vi "WILT.vi"() -> ()   [LabVIEW 2016] (continued)
            n368 = event-data() -> ("NewVal"=w742:bool)  [unwired: 1 in, 2 out]
            n369 = case shown="True" w742 {
              tunnel: w745 -> [_ w758]
              tunnel: w744 -> [w748 w756]
              tunnel: [w748 w755] -> w743
              tunnel: w742 -> [_ w753]
              frame False {
              }
              frame True {
                n370 = local read "Number of ON/OFF Cycles"() -> (w750:i32)
                n371 = local read "Valve ON Time (mS)"() -> (w749:u32)
                n372 = local read "Agilent Semaphore"() -> (w759:T1[])
                n373 = Unbundle By Name(w758) -> ("Agilent Switches"=w757:T2[])
                n374 = local read "Test Type"() -> (w751:T12)
                n375 = Number To Decimal String(number=32) -> (decimal integer string=w761:string)  [unwired: 1 in]
                n376 = Not(x=w753) -> (.not. x?=w760:bool)
                n377 = call "WILT Agilent Valve Control.vi"("Station In"=w761, "Agilent Channels In"=w757, "Semaphore"=w759, "Search"=T19 "Water Valve", "Open/Close (F:Close)"=w760, "error in (no error)"=w756, "Test Type"=w751, "Number Of Cycles"=w750, "Cycle Time (mS)"=w749) -> ("error out"=w755:errorcluster)  [unwired: 4 in, 2 out]
              }
            }
            n378 = call <vilib>:"Add State(s) to Queue__jki_lib_state_machine.vi"("State(s) in (\"\")"=w747) -> ("States Out"=w746:string)  [unwired: 14 in]
          }
          event Value Change {
            n379 = event-data() -> ("NewVal"=w762:bool)  [unwired: 1 in, 2 out]
            n380 = case shown="True" w762 {
              tunnel: w765 -> [_ w778]
              tunnel: w764 -> [w768 w776]
              tunnel: [w768 w775] -> w763
              tunnel: w762 -> [_ w773]
              frame False {
              }
              frame True {
                n381 = local read "Number of ON/OFF Cycles"() -> (w770:i32)
                n382 = local read "Valve ON Time (mS)"() -> (w769:u32)
                n383 = local read "Agilent Semaphore"() -> (w779:T1[])
                n384 = Unbundle By Name(w778) -> ("Agilent Switches"=w777:T2[])
                n385 = local read "Test Type"() -> (w771:T12)
                n386 = Number To Decimal String(number=33) -> (decimal integer string=w781:string)  [unwired: 1 in]
                n387 = Not(x=w773) -> (.not. x?=w780:bool)
                n388 = call "WILT Agilent Valve Control.vi"("Station In"=w781, "Agilent Channels In"=w777, "Semaphore"=w779, "Search"=T19 "Water Valve", "Open/Close (F:Close)"=w780, "error in (no error)"=w776, "Test Type"=w771, "Number Of Cycles"=w770, "Cycle Time (mS)"=w769) -> ("error out"=w775:errorcluster)  [unwired: 4 in, 2 out]
              }
            }
            n389 = call <vilib>:"Add State(s) to Queue__jki_lib_state_machine.vi"("State(s) in (\"\")"=w767) -> ("States Out"=w766:string)  [unwired: 14 in]
          }
          event Value Change {
            n390 = event-data() -> ("NewVal"=w782:bool)  [unwired: 1 in, 2 out]
            n391 = case shown="True" w782 {
              tunnel: w785 -> [_ w798]
              tunnel: w784 -> [w788 w796]
              tunnel: [w788 w795] -> w783
              tunnel: w782 -> [_ w793]
              frame False {
              }
              frame True {
                n392 = local read "Number of ON/OFF Cycles"() -> (w790:i32)
                n393 = local read "Valve ON Time (mS)"() -> (w789:u32)
                n394 = local read "Agilent Semaphore"() -> (w799:T1[])
                n395 = Unbundle By Name(w798) -> ("Agilent Switches"=w797:T2[])
                n396 = local read "Test Type"() -> (w791:T12)
                n397 = Number To Decimal String(number=34) -> (decimal integer string=w801:string)  [unwired: 1 in]
                n398 = Not(x=w793) -> (.not. x?=w800:bool)
                n399 = call "WILT Agilent Valve Control.vi"("Station In"=w801, "Agilent Channels In"=w797, "Semaphore"=w799, "Search"=T19 "Water Valve", "Open/Close (F:Close)"=w800, "error in (no error)"=w796, "Test Type"=w791, "Number Of Cycles"=w790, "Cycle Time (mS)"=w789) -> ("error out"=w795:errorcluster)  [unwired: 4 in, 2 out]
              }
            }
            n400 = call <vilib>:"Add State(s) to Queue__jki_lib_state_machine.vi"("State(s) in (\"\")"=w787) -> ("States Out"=w786:string)  [unwired: 14 in]
          }
          event Value Change {
            n401 = event-data() -> ("NewVal"=w802:bool)  [unwired: 1 in, 2 out]
            n402 = case shown="True" w802 {
              tunnel: w805 -> [_ w818]
              tunnel: w804 -> [w808 w816]
              tunnel: [w808 w815] -> w803
              tunnel: w802 -> [_ w813]
              frame False {
              }
              frame True {
                n403 = local read "Number of ON/OFF Cycles"() -> (w810:i32)
                n404 = local read "Valve ON Time (mS)"() -> (w809:u32)
                n405 = local read "Agilent Semaphore"() -> (w819:T1[])
                n406 = Unbundle By Name(w818) -> ("Agilent Switches"=w817:T2[])
                n407 = local read "Test Type"() -> (w811:T12)
                n408 = Number To Decimal String(number=35) -> (decimal integer string=w821:string)  [unwired: 1 in]
                n409 = Not(x=w813) -> (.not. x?=w820:bool)
                n410 = call "WILT Agilent Valve Control.vi"("Station In"=w821, "Agilent Channels In"=w817, "Semaphore"=w819, "Search"=T19 "Water Valve", "Open/Close (F:Close)"=w820, "error in (no error)"=w816, "Test Type"=w811, "Number Of Cycles"=w810, "Cycle Time (mS)"=w809) -> ("error out"=w815:errorcluster)  [unwired: 4 in, 2 out]
              }
            }
            n411 = call <vilib>:"Add State(s) to Queue__jki_lib_state_machine.vi"("State(s) in (\"\")"=w807) -> ("States Out"=w806:string)  [unwired: 14 in]
          }
          event Value Change {
            n412 = event-data() -> ("NewVal"=w822:bool)  [unwired: 1 in, 2 out]
            n413 = case shown="True" w822 {
              tunnel: w825 -> [_ w838]
              tunnel: w824 -> [w828 w836]
              tunnel: [w828 w835] -> w823
              tunnel: w822 -> [_ w833]
              frame False {
              }
              frame True {
                n414 = local read "Number of ON/OFF Cycles"() -> (w830:i32)
                n415 = local read "Valve ON Time (mS)"() -> (w829:u32)
                n416 = local read "Agilent Semaphore"() -> (w839:T1[])
                n417 = Unbundle By Name(w838) -> ("Agilent Switches"=w837:T2[])
                n418 = local read "Test Type"() -> (w831:T12)
                n419 = Number To Decimal String(number=36) -> (decimal integer string=w841:string)  [unwired: 1 in]
                n420 = Not(x=w833) -> (.not. x?=w840:bool)
                n421 = call "WILT Agilent Valve Control.vi"("Station In"=w841, "Agilent Channels In"=w837, "Semaphore"=w839, "Search"=T19 "Water Valve", "Open/Close (F:Close)"=w840, "error in (no error)"=w836, "Test Type"=w831, "Number Of Cycles"=w830, "Cycle Time (mS)"=w829) -> ("error out"=w835:errorcluster)  [unwired: 4 in, 2 out]
              }
            }
            n422 = call <vilib>:"Add State(s) to Queue__jki_lib_state_machine.vi"("State(s) in (\"\")"=w827) -> ("States Out"=w826:string)  [unwired: 14 in]
          }
          event Value Change {
            n423 = event-data() -> ("NewVal"=w842:bool)  [unwired: 1 in, 2 out]
            n424 = case shown="True" w842 {
              tunnel: w845 -> [_ w858]
              tunnel: w844 -> [w848 w856]
              tunnel: [w848 w855] -> w843
              tunnel: w842 -> [_ w853]
              frame False {
              }
              frame True {
                n425 = local read "Number of ON/OFF Cycles"() -> (w850:i32)
                n426 = local read "Valve ON Time (mS)"() -> (w849:u32)
                n427 = local read "Agilent Semaphore"() -> (w859:T1[])
                n428 = Unbundle By Name(w858) -> ("Agilent Switches"=w857:T2[])
                n429 = local read "Test Type"() -> (w851:T12)
                n430 = Number To Decimal String(number=37) -> (decimal integer string=w861:string)  [unwired: 1 in]
                n431 = Not(x=w853) -> (.not. x?=w860:bool)
                n432 = call "WILT Agilent Valve Control.vi"("Station In"=w861, "Agilent Channels In"=w857, "Semaphore"=w859, "Search"=T19 "Water Valve", "Open/Close (F:Close)"=w860, "error in (no error)"=w856, "Test Type"=w851, "Number Of Cycles"=w850, "Cycle Time (mS)"=w849) -> ("error out"=w855:errorcluster)  [unwired: 4 in, 2 out]
              }
            }
            n433 = call <vilib>:"Add State(s) to Queue__jki_lib_state_machine.vi"("State(s) in (\"\")"=w847) -> ("States Out"=w846:string)  [unwired: 14 in]
          }
          event Value Change {
            n434 = event-data() -> ("NewVal"=w862:bool)  [unwired: 1 in, 2 out]
            n435 = case shown="True" w862 {
              tunnel: w865 -> [_ w878]
              tunnel: w864 -> [w868 w876]
              tunnel: [w868 w875] -> w863
              tunnel: w862 -> [_ w873]
              frame False {
              }
              frame True {
                n436 = local read "Number of ON/OFF Cycles"() -> (w870:i32)
                n437 = local read "Valve ON Time (mS)"() -> (w869:u32)
                n438 = local read "Agilent Semaphore"() -> (w879:T1[])
                n439 = Unbundle By Name(w878) -> ("Agilent Switches"=w877:T2[])
                n440 = local read "Test Type"() -> (w871:T12)
                n441 = Number To Decimal String(number=38) -> (decimal integer string=w881:string)  [unwired: 1 in]
                n442 = Not(x=w873) -> (.not. x?=w880:bool)
                n443 = call "WILT Agilent Valve Control.vi"("Station In"=w881, "Agilent Channels In"=w877, "Semaphore"=w879, "Search"=T19 "Water Valve", "Open/Close (F:Close)"=w880, "error in (no error)"=w876, "Test Type"=w871, "Number Of Cycles"=w870, "Cycle Time (mS)"=w869) -> ("error out"=w875:errorcluster)  [unwired: 4 in, 2 out]
              }
            }
            n444 = call <vilib>:"Add State(s) to Queue__jki_lib_state_machine.vi"("State(s) in (\"\")"=w867) -> ("States Out"=w866:string)  [unwired: 14 in]
          }
          event Value Change {
            n445 = event-data() -> ("NewVal"=w882:bool)  [unwired: 1 in, 2 out]
            n446 = case shown="True" w882 {
              tunnel: w885 -> [_ w898]
              tunnel: w884 -> [w888 w896]
              tunnel: [w888 w895] -> w883
              tunnel: w882 -> [_ w893]
              frame False {
              }
              frame True {
                n447 = local read "Number of ON/OFF Cycles"() -> (w890:i32)
                n448 = local read "Valve ON Time (mS)"() -> (w889:u32)
                n449 = local read "Agilent Semaphore"() -> (w899:T1[])
                n450 = Unbundle By Name(w898) -> ("Agilent Switches"=w897:T2[])
                n451 = local read "Test Type"() -> (w891:T12)
                n452 = Number To Decimal String(number=39) -> (decimal integer string=w901:string)  [unwired: 1 in]
                n453 = Not(x=w893) -> (.not. x?=w900:bool)
                n454 = call "WILT Agilent Valve Control.vi"("Station In"=w901, "Agilent Channels In"=w897, "Semaphore"=w899, "Search"=T19 "Water Valve", "Open/Close (F:Close)"=w900, "error in (no error)"=w896, "Test Type"=w891, "Number Of Cycles"=w890, "Cycle Time (mS)"=w889) -> ("error out"=w895:errorcluster)  [unwired: 4 in, 2 out]
              }
            }
            n455 = call <vilib>:"Add State(s) to Queue__jki_lib_state_machine.vi"("State(s) in (\"\")"=w887) -> ("States Out"=w886:string)  [unwired: 14 in]
          }
          event Value Change {
            n456 = event-data() -> ("NewVal"=w902:bool)  [unwired: 1 in, 2 out]
            n457 = case shown="True" w902 {
              tunnel: w905 -> [_ w918]
              tunnel: w904 -> [w908 w916]
              tunnel: [w908 w915] -> w903
              tunnel: w902 -> [_ w913]
              frame False {
              }
              frame True {
                n458 = local read "Number of ON/OFF Cycles"() -> (w910:i32)
                n459 = local read "Valve ON Time (mS)"() -> (w909:u32)
                n460 = local read "Agilent Semaphore"() -> (w919:T1[])
                n461 = Unbundle By Name(w918) -> ("Agilent Switches"=w917:T2[])
                n462 = local read "Test Type"() -> (w911:T12)
                n463 = Number To Decimal String(number=40) -> (decimal integer string=w921:string)  [unwired: 1 in]
                n464 = Not(x=w913) -> (.not. x?=w920:bool)
                n465 = call "WILT Agilent Valve Control.vi"("Station In"=w921, "Agilent Channels In"=w917, "Semaphore"=w919, "Search"=T19 "Water Valve", "Open/Close (F:Close)"=w920, "error in (no error)"=w916, "Test Type"=w911, "Number Of Cycles"=w910, "Cycle Time (mS)"=w909) -> ("error out"=w915:errorcluster)  [unwired: 4 in, 2 out]
              }
            }
            n466 = call <vilib>:"Add State(s) to Queue__jki_lib_state_machine.vi"("State(s) in (\"\")"=w907) -> ("States Out"=w906:string)  [unwired: 14 in]
          }
          event Value Change {
            n467 = event-data() -> ("NewVal"=w922:bool)  [unwired: 1 in, 2 out]
            n468 = case shown="False" w922 {
              tunnel: w925 -> [_ w938]
              tunnel: w924 -> [w928 w936]
              tunnel: [w928 w935] -> w923
              tunnel: w922 -> [_ w933]
              frame False {
              }
              frame True {
                n469 = local read "Number of ON/OFF Cycles"() -> (w930:i32)
                n470 = local read "Valve ON Time (mS)"() -> (w929:u32)
                n471 = local read "Agilent Semaphore"() -> (w939:T1[])
                n472 = Unbundle By Name(w938) -> ("Agilent Switches"=w937:T2[])
                n473 = local read "Test Type"() -> (w931:T12)
                n474 = Number To Decimal String(number=41) -> (decimal integer string=w941:string)  [unwired: 1 in]
                n475 = Not(x=w933) -> (.not. x?=w940:bool)
                n476 = call "WILT Agilent Valve Control.vi"("Station In"=w941, "Agilent Channels In"=w937, "Semaphore"=w939, "Search"=T19 "Water Valve", "Open/Close (F:Close)"=w940, "error in (no error)"=w936, "Test Type"=w931, "Number Of Cycles"=w930, "Cycle Time (mS)"=w929) -> ("error out"=w935:errorcluster)  [unwired: 4 in, 2 out]
              }
            }
            n477 = call <vilib>:"Add State(s) to Queue__jki_lib_state_machine.vi"("State(s) in (\"\")"=w927) -> ("States Out"=w926:string)  [unwired: 14 in]
          }
          event Value Change {
            n478 = event-data() -> ("NewVal"=w942:bool)  [unwired: 1 in, 2 out]
            n479 = case shown="True" w942 {
              tunnel: w945 -> [_ w958]
              tunnel: w944 -> [w948 w956]
              tunnel: [w948 w955] -> w943
              tunnel: w942 -> [_ w953]
              frame False {
              }
              frame True {
                n480 = local read "Number of ON/OFF Cycles"() -> (w950:i32)
                n481 = local read "Valve ON Time (mS)"() -> (w949:u32)
                n482 = local read "Agilent Semaphore"() -> (w959:T1[])
                n483 = Unbundle By Name(w958) -> ("Agilent Switches"=w957:T2[])
                n484 = local read "Test Type"() -> (w951:T12)
                n485 = Number To Decimal String(number=42) -> (decimal integer string=w961:string)  [unwired: 1 in]
                n486 = Not(x=w953) -> (.not. x?=w960:bool)
                n487 = call "WILT Agilent Valve Control.vi"("Station In"=w961, "Agilent Channels In"=w957, "Semaphore"=w959, "Search"=T19 "Water Valve", "Open/Close (F:Close)"=w960, "error in (no error)"=w956, "Test Type"=w951, "Number Of Cycles"=w950, "Cycle Time (mS)"=w949) -> ("error out"=w955:errorcluster)  [unwired: 4 in, 2 out]
              }
            }
            n488 = call <vilib>:"Add State(s) to Queue__jki_lib_state_machine.vi"("State(s) in (\"\")"=w947) -> ("States Out"=w946:string)  [unwired: 14 in]
          }
          event Value Change {
            n489 = event-data() -> ("NewVal"=w962:bool)  [unwired: 1 in, 2 out]
            n490 = case shown="True" w962 {
              tunnel: w965 -> [_ w978]
              tunnel: w964 -> [w968 w976]
              tunnel: [w968 w975] -> w963
              tunnel: w962 -> [_ w973]
              frame False {
              }
              frame True {
                n491 = local read "Number of ON/OFF Cycles"() -> (w970:i32)
                n492 = local read "Valve ON Time (mS)"() -> (w969:u32)
                n493 = local read "Agilent Semaphore"() -> (w979:T1[])
                n494 = Unbundle By Name(w978) -> ("Agilent Switches"=w977:T2[])
                n495 = local read "Test Type"() -> (w971:T12)
                n496 = Number To Decimal String(number=43) -> (decimal integer string=w981:string)  [unwired: 1 in]
                n497 = Not(x=w973) -> (.not. x?=w980:bool)
                n498 = call "WILT Agilent Valve Control.vi"("Station In"=w981, "Agilent Channels In"=w977, "Semaphore"=w979, "Search"=T19 "Water Valve", "Open/Close (F:Close)"=w980, "error in (no error)"=w976, "Test Type"=w971, "Number Of Cycles"=w970, "Cycle Time (mS)"=w969) -> ("error out"=w975:errorcluster)  [unwired: 4 in, 2 out]
              }
            }
            n499 = call <vilib>:"Add State(s) to Queue__jki_lib_state_machine.vi"("State(s) in (\"\")"=w967) -> ("States Out"=w966:string)  [unwired: 14 in]
          }
          event Value Change {
            n500 = event-data() -> ("NewVal"=w982:bool)  [unwired: 1 in, 2 out]
            n501 = case shown="True" w982 {
              tunnel: w985 -> [_ w998]
              tunnel: w984 -> [w988 w996]
              tunnel: [w988 w995] -> w983
              tunnel: w982 -> [_ w993]
              frame False {
              }
              frame True {
                n502 = local read "Number of ON/OFF Cycles"() -> (w990:i32)
                n503 = local read "Valve ON Time (mS)"() -> (w989:u32)
                n504 = local read "Agilent Semaphore"() -> (w999:T1[])
                n505 = Unbundle By Name(w998) -> ("Agilent Switches"=w997:T2[])
                n506 = local read "Test Type"() -> (w991:T12)
                n507 = Number To Decimal String(number=44) -> (decimal integer string=w1001:string)  [unwired: 1 in]
                n508 = Not(x=w993) -> (.not. x?=w1000:bool)
                n509 = call "WILT Agilent Valve Control.vi"("Station In"=w1001, "Agilent Channels In"=w997, "Semaphore"=w999, "Search"=T19 "Water Valve", "Open/Close (F:Close)"=w1000, "error in (no error)"=w996, "Test Type"=w991, "Number Of Cycles"=w990, "Cycle Time (mS)"=w989) -> ("error out"=w995:errorcluster)  [unwired: 4 in, 2 out]
              }
            }
            n510 = call <vilib>:"Add State(s) to Queue__jki_lib_state_machine.vi"("State(s) in (\"\")"=w987) -> ("States Out"=w986:string)  [unwired: 14 in]
          }
          event Value Change {
            n511 = event-data() -> ("NewVal"=w1002:bool)  [unwired: 1 in, 2 out]
            n512 = case shown="False" w1002 {
              tunnel: w1005 -> [_ w1018]
              tunnel: w1004 -> [w1008 w1016]
              tunnel: [w1008 w1015] -> w1003
              tunnel: w1002 -> [_ w1013]
              frame False {
              }
              frame True {
                n513 = local read "Number of ON/OFF Cycles"() -> (w1010:i32)
                n514 = local read "Valve ON Time (mS)"() -> (w1009:u32)
                n515 = local read "Agilent Semaphore"() -> (w1019:T1[])
                n516 = Unbundle By Name(w1018) -> ("Agilent Switches"=w1017:T2[])
                n517 = local read "Test Type"() -> (w1011:T12)
                n518 = Number To Decimal String(number=45) -> (decimal integer string=w1021:string)  [unwired: 1 in]
                n519 = Not(x=w1013) -> (.not. x?=w1020:bool)
                n520 = call "WILT Agilent Valve Control.vi"("Station In"=w1021, "Agilent Channels In"=w1017, "Semaphore"=w1019, "Search"=T19 "Water Valve", "Open/Close (F:Close)"=w1020, "error in (no error)"=w1016, "Test Type"=w1011, "Number Of Cycles"=w1010, "Cycle Time (mS)"=w1009) -> ("error out"=w1015:errorcluster)  [unwired: 4 in, 2 out]
              }
            }
            n521 = call <vilib>:"Add State(s) to Queue__jki_lib_state_machine.vi"("State(s) in (\"\")"=w1007) -> ("States Out"=w1006:string)  [unwired: 14 in]
          }
          event Value Change {
            n522 = event-data() -> ("NewVal"=w1022:bool)  [unwired: 1 in, 2 out]
            n523 = case shown="True" w1022 {
              tunnel: w1025 -> [_ w1038]
              tunnel: w1024 -> [w1028 w1036]
              tunnel: [w1028 w1035] -> w1023
              tunnel: w1022 -> [_ w1033]
              frame False {
              }
              frame True {
                n524 = local read "Number of ON/OFF Cycles"() -> (w1030:i32)
                n525 = local read "Valve ON Time (mS)"() -> (w1029:u32)
                n526 = local read "Agilent Semaphore"() -> (w1039:T1[])
                n527 = Unbundle By Name(w1038) -> ("Agilent Switches"=w1037:T2[])
                n528 = local read "Test Type"() -> (w1031:T12)
                n529 = Number To Decimal String(number=46) -> (decimal integer string=w1041:string)  [unwired: 1 in]
                n530 = Not(x=w1033) -> (.not. x?=w1040:bool)
                n531 = call "WILT Agilent Valve Control.vi"("Station In"=w1041, "Agilent Channels In"=w1037, "Semaphore"=w1039, "Search"=T19 "Water Valve", "Open/Close (F:Close)"=w1040, "error in (no error)"=w1036, "Test Type"=w1031, "Number Of Cycles"=w1030, "Cycle Time (mS)"=w1029) -> ("error out"=w1035:errorcluster)  [unwired: 4 in, 2 out]
              }
            }
            n532 = call <vilib>:"Add State(s) to Queue__jki_lib_state_machine.vi"("State(s) in (\"\")"=w1027) -> ("States Out"=w1026:string)  [unwired: 14 in]
          }
          event Value Change {
            n533 = event-data() -> ("NewVal"=w1042:bool)  [unwired: 1 in, 2 out]
            n534 = case shown="True" w1042 {
              tunnel: w1045 -> [_ w1058]
              tunnel: w1044 -> [w1048 w1056]
              tunnel: [w1048 w1055] -> w1043
              tunnel: w1042 -> [_ w1053]
              frame False {
              }
              frame True {
                n535 = local read "Number of ON/OFF Cycles"() -> (w1050:i32)
                n536 = local read "Agilent Semaphore"() -> (w1059:T1[])
                n537 = local read "Valve ON Time (mS)"() -> (w1049:u32)
                n538 = Unbundle By Name(w1058) -> ("Agilent Switches"=w1057:T2[])
                n539 = local read "Test Type"() -> (w1051:T12)
                n540 = Number To Decimal String(number=47) -> (decimal integer string=w1061:string)  [unwired: 1 in]
                n541 = Not(x=w1053) -> (.not. x?=w1060:bool)
                n542 = call "WILT Agilent Valve Control.vi"("Station In"=w1061, "Agilent Channels In"=w1057, "Semaphore"=w1059, "Search"=T19 "Water Valve", "Open/Close (F:Close)"=w1060, "error in (no error)"=w1056, "Test Type"=w1051, "Number Of Cycles"=w1050, "Cycle Time (mS)"=w1049) -> ("error out"=w1055:errorcluster)  [unwired: 4 in, 2 out]
              }
            }
            n543 = call <vilib>:"Add State(s) to Queue__jki_lib_state_machine.vi"("State(s) in (\"\")"=w1047) -> ("States Out"=w1046:string)  [unwired: 14 in]
          }
          event Value Change {
            n544 = event-data() -> ("NewVal"=w1062:bool)  [unwired: 1 in, 2 out]
            n545 = case shown="True" w1062 {
              tunnel: w1065 -> [_ w1078]
              tunnel: w1064 -> [w1068 w1076]
              tunnel: [w1068 w1075] -> w1063
              tunnel: w1062 -> [_ w1073]
              frame False {
              }
              frame True {
                n546 = local read "Number of ON/OFF Cycles"() -> (w1070:i32)
                n547 = local read "Valve ON Time (mS)"() -> (w1069:u32)
                n548 = local read "Agilent Semaphore"() -> (w1079:T1[])
                n549 = Unbundle By Name(w1078) -> ("Agilent Switches"=w1077:T2[])
                n550 = local read "Test Type"() -> (w1071:T12)
                n551 = Number To Decimal String(number=48) -> (decimal integer string=w1081:string)  [unwired: 1 in]
                n552 = Not(x=w1073) -> (.not. x?=w1080:bool)
                n553 = call "WILT Agilent Valve Control.vi"("Station In"=w1081, "Agilent Channels In"=w1077, "Semaphore"=w1079, "Search"=T19 "Water Valve", "Open/Close (F:Close)"=w1080, "error in (no error)"=w1076, "Test Type"=w1071, "Number Of Cycles"=w1070, "Cycle Time (mS)"=w1069) -> ("error out"=w1075:errorcluster)  [unwired: 4 in, 2 out]
              }
            }
            n554 = call <vilib>:"Add State(s) to Queue__jki_lib_state_machine.vi"("State(s) in (\"\")"=w1067) -> ("States Out"=w1066:string)  [unwired: 14 in]
          }
          event Value Change {
            n555 = event-data() -> ("NewVal"=w1082:bool)  [unwired: 1 in, 2 out]
            n556 = case shown="False" w1082 {
              tunnel: w1085 -> [_ w1098]
              tunnel: w1084 -> [w1088 w1096]
              tunnel: [w1088 w1095] -> w1083
              tunnel: w1082 -> [_ w1093]
              frame False {
              }
              frame True {
                n557 = local read "Number of ON/OFF Cycles"() -> (w1090:i32)
                n558 = local read "Valve ON Time (mS)"() -> (w1089:u32)
                n559 = local read "Agilent Semaphore"() -> (w1099:T1[])
                n560 = Unbundle By Name(w1098) -> ("Agilent Switches"=w1097:T2[])
                n561 = local read "Test Type"() -> (w1091:T12)
                n562 = Number To Decimal String(number=49) -> (decimal integer string=w1101:string)  [unwired: 1 in]
                n563 = Not(x=w1093) -> (.not. x?=w1100:bool)
                n564 = call "WILT Agilent Valve Control.vi"("Station In"=w1101, "Agilent Channels In"=w1097, "Semaphore"=w1099, "Search"=T19 "Water Valve", "Open/Close (F:Close)"=w1100, "error in (no error)"=w1096, "Test Type"=w1091, "Number Of Cycles"=w1090, "Cycle Time (mS)"=w1089) -> ("error out"=w1095:errorcluster)  [unwired: 4 in, 2 out]
              }
            }
            n565 = call <vilib>:"Add State(s) to Queue__jki_lib_state_machine.vi"("State(s) in (\"\")"=w1087) -> ("States Out"=w1086:string)  [unwired: 14 in]
          }
          event Value Change {
            n566 = event-data() -> ("NewVal"=w1102:bool)  [unwired: 1 in, 2 out]
            n567 = case shown="False" w1102 {
              tunnel: w1105 -> [_ w1118]
              tunnel: w1104 -> [w1108 w1116]
              tunnel: [w1108 w1115] -> w1103
              tunnel: w1102 -> [_ w1113]
              frame False {
              }
              frame True {
                n568 = local read "Number of ON/OFF Cycles"() -> (w1110:i32)
                n569 = local read "Valve ON Time (mS)"() -> (w1109:u32)
                n570 = local read "Agilent Semaphore"() -> (w1119:T1[])
                n571 = Unbundle By Name(w1118) -> ("Agilent Switches"=w1117:T2[])
                n572 = local read "Test Type"() -> (w1111:T12)
                n573 = Number To Decimal String(number=50) -> (decimal integer string=w1121:string)  [unwired: 1 in]
                n574 = Not(x=w1113) -> (.not. x?=w1120:bool)
                n575 = call "WILT Agilent Valve Control.vi"("Station In"=w1121, "Agilent Channels In"=w1117, "Semaphore"=w1119, "Search"=T19 "Water Valve", "Open/Close (F:Close)"=w1120, "error in (no error)"=w1116, "Test Type"=w1111, "Number Of Cycles"=w1110, "Cycle Time (mS)"=w1109) -> ("error out"=w1115:errorcluster)  [unwired: 4 in, 2 out]
              }
            }
            n576 = call <vilib>:"Add State(s) to Queue__jki_lib_state_machine.vi"("State(s) in (\"\")"=w1107) -> ("States Out"=w1106:string)  [unwired: 14 in]
          }
          event Value Change {
            n577 = event-data() -> ("NewVal"=w1122:bool)  [unwired: 1 in, 2 out]
            n578 = case shown="True" w1122 {
              tunnel: w1125 -> [_ w1138]
              tunnel: w1124 -> [w1128 w1136]
              tunnel: [w1128 w1135] -> w1123
              tunnel: w1122 -> [_ w1133]
              frame False {
              }
              frame True {
                n579 = local read "Number of ON/OFF Cycles"() -> (w1130:i32)
                n580 = local read "Valve ON Time (mS)"() -> (w1129:u32)
                n581 = local read "Agilent Semaphore"() -> (w1139:T1[])
                n582 = Unbundle By Name(w1138) -> ("Agilent Switches"=w1137:T2[])
                n583 = local read "Test Type"() -> (w1131:T12)
                n584 = Number To Decimal String(number=51) -> (decimal integer string=w1141:string)  [unwired: 1 in]
                n585 = Not(x=w1133) -> (.not. x?=w1140:bool)
                n586 = call "WILT Agilent Valve Control.vi"("Station In"=w1141, "Agilent Channels In"=w1137, "Semaphore"=w1139, "Search"=T19 "Water Valve", "Open/Close (F:Close)"=w1140, "error in (no error)"=w1136, "Test Type"=w1131, "Number Of Cycles"=w1130, "Cycle Time (mS)"=w1129) -> ("error out"=w1135:errorcluster)  [unwired: 4 in, 2 out]
              }
            }
            n587 = call <vilib>:"Add State(s) to Queue__jki_lib_state_machine.vi"("State(s) in (\"\")"=w1127) -> ("States Out"=w1126:string)  [unwired: 14 in]
          }
          event Value Change {
            n588 = event-data() -> ("NewVal"=w1142:bool)  [unwired: 1 in, 2 out]
            n589 = case shown="True" w1142 {
              tunnel: w1145 -> [_ w1158]
              tunnel: w1144 -> [w1148 w1156]
              tunnel: [w1148 w1155] -> w1143
              tunnel: w1142 -> [_ w1153]
              frame False {
              }
              frame True {
                n590 = local read "Number of ON/OFF Cycles"() -> (w1150:i32)
                n591 = local read "Agilent Semaphore"() -> (w1159:T1[])
                n592 = local read "Valve ON Time (mS)"() -> (w1149:u32)
                n593 = Unbundle By Name(w1158) -> ("Agilent Switches"=w1157:T2[])
                n594 = local read "Test Type"() -> (w1151:T12)
                n595 = Number To Decimal String(number=52) -> (decimal integer string=w1161:string)  [unwired: 1 in]
                n596 = Not(x=w1153) -> (.not. x?=w1160:bool)
                n597 = call "WILT Agilent Valve Control.vi"("Station In"=w1161, "Agilent Channels In"=w1157, "Semaphore"=w1159, "Search"=T19 "Water Valve", "Open/Close (F:Close)"=w1160, "error in (no error)"=w1156, "Test Type"=w1151, "Number Of Cycles"=w1150, "Cycle Time (mS)"=w1149) -> ("error out"=w1155:errorcluster)  [unwired: 4 in, 2 out]
              }
            }
            n598 = call <vilib>:"Add State(s) to Queue__jki_lib_state_machine.vi"("State(s) in (\"\")"=w1147) -> ("States Out"=w1146:string)  [unwired: 14 in]
          }
          event Value Change {
            n599 = event-data() -> ("NewVal"=w1162:bool)  [unwired: 1 in, 2 out]
            n600 = case shown="True" w1162 {
              tunnel: w1165 -> [_ w1178]
              tunnel: w1164 -> [w1168 w1176]
              tunnel: [w1168 w1175] -> w1163
              tunnel: w1162 -> [_ w1173]
              frame False {
              }
              frame True {
                n601 = local read "Number of ON/OFF Cycles"() -> (w1170:i32)
                n602 = local read "Agilent Semaphore"() -> (w1179:T1[])
                n603 = local read "Valve ON Time (mS)"() -> (w1169:u32)
                n604 = Unbundle By Name(w1178) -> ("Agilent Switches"=w1177:T2[])
                n605 = local read "Test Type"() -> (w1171:T12)
                n606 = Number To Decimal String(number=53) -> (decimal integer string=w1181:string)  [unwired: 1 in]
                n607 = Not(x=w1173) -> (.not. x?=w1180:bool)
                n608 = call "WILT Agilent Valve Control.vi"("Station In"=w1181, "Agilent Channels In"=w1177, "Semaphore"=w1179, "Search"=T19 "Water Valve", "Open/Close (F:Close)"=w1180, "error in (no error)"=w1176, "Test Type"=w1171, "Number Of Cycles"=w1170, "Cycle Time (mS)"=w1169) -> ("error out"=w1175:errorcluster)  [unwired: 4 in, 2 out]
              }
            }
            n609 = call <vilib>:"Add State(s) to Queue__jki_lib_state_machine.vi"("State(s) in (\"\")"=w1167) -> ("States Out"=w1166:string)  [unwired: 14 in]
          }
          event Value Change {
            n610 = event-data() -> ("NewVal"=w1182:bool)  [unwired: 1 in, 2 out]
            n611 = case shown="True" w1182 {
              tunnel: w1185 -> [_ w1198]
              tunnel: w1184 -> [w1188 w1196]
              tunnel: [w1188 w1195] -> w1183
              tunnel: w1182 -> [_ w1193]
              frame False {
              }
              frame True {
                n612 = local read "Number of ON/OFF Cycles"() -> (w1190:i32)
                n613 = local read "Agilent Semaphore"() -> (w1199:T1[])
                n614 = Unbundle By Name(w1198) -> ("Agilent Switches"=w1197:T2[])
                n615 = local read "Valve ON Time (mS)"() -> (w1189:u32)
                n616 = local read "Test Type"() -> (w1191:T12)
                n617 = Number To Decimal String(number=54) -> (decimal integer string=w1201:string)  [unwired: 1 in]
                n618 = Not(x=w1193) -> (.not. x?=w1200:bool)
                n619 = call "WILT Agilent Valve Control.vi"("Station In"=w1201, "Agilent Channels In"=w1197, "Semaphore"=w1199, "Search"=T19 "Water Valve", "Open/Close (F:Close)"=w1200, "error in (no error)"=w1196, "Test Type"=w1191, "Number Of Cycles"=w1190, "Cycle Time (mS)"=w1189) -> ("error out"=w1195:errorcluster)  [unwired: 4 in, 2 out]
              }
            }
            n620 = call <vilib>:"Add State(s) to Queue__jki_lib_state_machine.vi"("State(s) in (\"\")"=w1187) -> ("States Out"=w1186:string)  [unwired: 14 in]
          }
          event Value Change {
            n621 = event-data() -> ("NewVal"=w1202:bool)  [unwired: 1 in, 2 out]
            n622 = case shown="True" w1202 {
              tunnel: w1205 -> [_ w1218]
              tunnel: w1204 -> [w1208 w1216]
              tunnel: [w1208 w1215] -> w1203
              tunnel: w1202 -> [_ w1213]
              frame False {
              }
              frame True {
                n623 = local read "Number of ON/OFF Cycles"() -> (w1210:i32)
                n624 = local read "Agilent Semaphore"() -> (w1219:T1[])
                n625 = local read "Valve ON Time (mS)"() -> (w1209:u32)
                n626 = Unbundle By Name(w1218) -> ("Agilent Switches"=w1217:T2[])
                n627 = local read "Test Type"() -> (w1211:T12)
                n628 = Number To Decimal String(number=55) -> (decimal integer string=w1221:string)  [unwired: 1 in]
                n629 = Not(x=w1213) -> (.not. x?=w1220:bool)
                n630 = call "WILT Agilent Valve Control.vi"("Station In"=w1221, "Agilent Channels In"=w1217, "Semaphore"=w1219, "Search"=T19 "Water Valve", "Open/Close (F:Close)"=w1220, "error in (no error)"=w1216, "Test Type"=w1211, "Number Of Cycles"=w1210, "Cycle Time (mS)"=w1209) -> ("error out"=w1215:errorcluster)  [unwired: 4 in, 2 out]
              }
            }
            n631 = call <vilib>:"Add State(s) to Queue__jki_lib_state_machine.vi"("State(s) in (\"\")"=w1207) -> ("States Out"=w1206:string)  [unwired: 14 in]
          }
          event Value Change {
            n632 = event-data() -> ("NewVal"=w1222:bool)  [unwired: 1 in, 2 out]
            n633 = case shown="True" w1222 {
              tunnel: w1225 -> [_ w1238]
              tunnel: w1224 -> [w1228 w1236]
              tunnel: [w1228 w1235] -> w1223
              tunnel: w1222 -> [_ w1233]
              frame False {
              }
              frame True {
                n634 = local read "Number of ON/OFF Cycles"() -> (w1230:i32)
                n635 = local read "Valve ON Time (mS)"() -> (w1229:u32)
                n636 = local read "Agilent Semaphore"() -> (w1239:T1[])
                n637 = Unbundle By Name(w1238) -> ("Agilent Switches"=w1237:T2[])
                n638 = local read "Test Type"() -> (w1231:T12)
                n639 = Number To Decimal String(number=56) -> (decimal integer string=w1241:string)  [unwired: 1 in]
                n640 = Not(x=w1233) -> (.not. x?=w1240:bool)
                n641 = call "WILT Agilent Valve Control.vi"("Station In"=w1241, "Agilent Channels In"=w1237, "Semaphore"=w1239, "Search"=T19 "Water Valve", "Open/Close (F:Close)"=w1240, "error in (no error)"=w1236, "Test Type"=w1231, "Number Of Cycles"=w1230, "Cycle Time (mS)"=w1229) -> ("error out"=w1235:errorcluster)  [unwired: 4 in, 2 out]
              }
            }
            n642 = call <vilib>:"Add State(s) to Queue__jki_lib_state_machine.vi"("State(s) in (\"\")"=w1227) -> ("States Out"=w1226:string)  [unwired: 14 in]
          }
          event Value Change {
            n643 = event-data() -> ("NewVal"=w1242:bool)  [unwired: 1 in, 2 out]
            n644 = case shown="True" w1242 {
              tunnel: w1245 -> [_ w1258]
              tunnel: w1244 -> [w1248 w1256]
              tunnel: [w1248 w1255] -> w1243
              tunnel: w1242 -> [_ w1253]
              frame False {
              }
              frame True {
                n645 = local read "Number of ON/OFF Cycles"() -> (w1250:i32)
                n646 = local read "Valve ON Time (mS)"() -> (w1249:u32)
                n647 = local read "Agilent Semaphore"() -> (w1259:T1[])
                n648 = Unbundle By Name(w1258) -> ("Agilent Switches"=w1257:T2[])
                n649 = local read "Test Type"() -> (w1251:T12)
                n650 = Number To Decimal String(number=1) -> (decimal integer string=w1261:string)  [unwired: 1 in]
                n651 = Not(x=w1253) -> (.not. x?=w1260:bool)
                n652 = call "WILT Agilent Valve Control.vi"("Station In"=w1261, "Agilent Channels In"=w1257, "Semaphore"=w1259, "Search"=T19 "Start Button", "Open/Close (F:Close)"=w1260, "error in (no error)"=w1256, "Test Type"=w1251, "Number Of Cycles"=w1250, "Cycle Time (mS)"=w1249) -> ("error out"=w1255:errorcluster)  [unwired: 4 in, 2 out]
              }
            }
            n653 = call <vilib>:"Add State(s) to Queue__jki_lib_state_machine.vi"("State(s) in (\"\")"=w1247) -> ("States Out"=w1246:string)  [unwired: 14 in]
          }
          event Value Change {
            n654 = event-data() -> ("NewVal"=w1262:bool)  [unwired: 1 in, 2 out]
            n655 = case shown="True" w1262 {
              tunnel: w1265 -> [_ w1278]
              tunnel: w1264 -> [w1268 w1276]
              tunnel: [w1268 w1275] -> w1263
              tunnel: w1262 -> [_ w1273]
              frame False {
              }
              frame True {
                n656 = local read "Number of ON/OFF Cycles"() -> (w1270:i32)
                n657 = local read "Valve ON Time (mS)"() -> (w1269:u32)
                n658 = local read "Agilent Semaphore"() -> (w1279:T1[])
                n659 = Unbundle By Name(w1278) -> ("Agilent Switches"=w1277:T2[])
                n660 = local read "Test Type"() -> (w1271:T12)
                n661 = Number To Decimal String(number=2) -> (decimal integer string=w1281:string)  [unwired: 1 in]
                n662 = Not(x=w1273) -> (.not. x?=w1280:bool)
                n663 = call "WILT Agilent Valve Control.vi"("Station In"=w1281, "Agilent Channels In"=w1277, "Semaphore"=w1279, "Search"=T19 "Start Button", "Open/Close (F:Close)"=w1280, "error in (no error)"=w1276, "Test Type"=w1271, "Number Of Cycles"=w1270, "Cycle Time (mS)"=w1269) -> ("error out"=w1275:errorcluster)  [unwired: 4 in, 2 out]
              }
            }
            n664 = call <vilib>:"Add State(s) to Queue__jki_lib_state_machine.vi"("State(s) in (\"\")"=w1267) -> ("States Out"=w1266:string)  [unwired: 14 in]
          }
          event Value Change {
            n665 = event-data() -> ("NewVal"=w1282:bool)  [unwired: 1 in, 2 out]
            n666 = case shown="True" w1282 {
              tunnel: w1285 -> [_ w1298]
              tunnel: w1284 -> [w1288 w1296]
              tunnel: [w1288 w1295] -> w1283
              tunnel: w1282 -> [_ w1293]
              frame False {
              }
              frame True {
                n667 = local read "Number of ON/OFF Cycles"() -> (w1290:i32)
                n668 = local read "Valve ON Time (mS)"() -> (w1289:u32)
                n669 = local read "Agilent Semaphore"() -> (w1299:T1[])
                n670 = Unbundle By Name(w1298) -> ("Agilent Switches"=w1297:T2[])
                n671 = local read "Test Type"() -> (w1291:T12)
                n672 = Number To Decimal String(number=3) -> (decimal integer string=w1301:string)  [unwired: 1 in]
                n673 = Not(x=w1293) -> (.not. x?=w1300:bool)
                n674 = call "WILT Agilent Valve Control.vi"("Station In"=w1301, "Agilent Channels In"=w1297, "Semaphore"=w1299, "Search"=T19 "Start Button", "Open/Close (F:Close)"=w1300, "error in (no error)"=w1296, "Test Type"=w1291, "Number Of Cycles"=w1290, "Cycle Time (mS)"=w1289) -> ("error out"=w1295:errorcluster)  [unwired: 4 in, 2 out]
              }
            }
            n675 = call <vilib>:"Add State(s) to Queue__jki_lib_state_machine.vi"("State(s) in (\"\")"=w1287) -> ("States Out"=w1286:string)  [unwired: 14 in]
          }
          event Value Change {
            n676 = event-data() -> ("NewVal"=w1302:bool)  [unwired: 1 in, 2 out]
            n677 = case shown="False" w1302 {
              tunnel: w1305 -> [_ w1318]
              tunnel: w1304 -> [w1308 w1316]
              tunnel: [w1308 w1315] -> w1303
              tunnel: w1302 -> [_ w1313]
              frame False {
              }
              frame True {
                n678 = local read "Number of ON/OFF Cycles"() -> (w1310:i32)
                n679 = local read "Valve ON Time (mS)"() -> (w1309:u32)
                n680 = local read "Agilent Semaphore"() -> (w1319:T1[])
                n681 = Unbundle By Name(w1318) -> ("Agilent Switches"=w1317:T2[])
                n682 = local read "Test Type"() -> (w1311:T12)
                n683 = Number To Decimal String(number=4) -> (decimal integer string=w1321:string)  [unwired: 1 in]
                n684 = Not(x=w1313) -> (.not. x?=w1320:bool)
                n685 = call "WILT Agilent Valve Control.vi"("Station In"=w1321, "Agilent Channels In"=w1317, "Semaphore"=w1319, "Search"=T19 "Start Button", "Open/Close (F:Close)"=w1320, "error in (no error)"=w1316, "Test Type"=w1311, "Number Of Cycles"=w1310, "Cycle Time (mS)"=w1309) -> ("error out"=w1315:errorcluster)  [unwired: 4 in, 2 out]
              }
            }
            n686 = call <vilib>:"Add State(s) to Queue__jki_lib_state_machine.vi"("State(s) in (\"\")"=w1307) -> ("States Out"=w1306:string)  [unwired: 14 in]
          }
          event Value Change {
            n687 = event-data() -> ("NewVal"=w1322:bool)  [unwired: 1 in, 2 out]
            n688 = case shown="False" w1322 {
              tunnel: w1325 -> [_ w1338]
              tunnel: w1324 -> [w1328 w1336]
              tunnel: [w1328 w1335] -> w1323
              tunnel: w1322 -> [_ w1333]
              frame False {
              }
              frame True {
                n689 = local read "Number of ON/OFF Cycles"() -> (w1330:i32)
                n690 = local read "Valve ON Time (mS)"() -> (w1329:u32)
                n691 = local read "Agilent Semaphore"() -> (w1339:T1[])
                n692 = Unbundle By Name(w1338) -> ("Agilent Switches"=w1337:T2[])
                n693 = local read "Test Type"() -> (w1331:T12)
                n694 = Number To Decimal String(number=5) -> (decimal integer string=w1341:string)  [unwired: 1 in]
                n695 = Not(x=w1333) -> (.not. x?=w1340:bool)
                n696 = call "WILT Agilent Valve Control.vi"("Station In"=w1341, "Agilent Channels In"=w1337, "Semaphore"=w1339, "Search"=T19 "Start Button", "Open/Close (F:Close)"=w1340, "error in (no error)"=w1336, "Test Type"=w1331, "Number Of Cycles"=w1330, "Cycle Time (mS)"=w1329) -> ("error out"=w1335:errorcluster)  [unwired: 4 in, 2 out]
              }
            }
            n697 = call <vilib>:"Add State(s) to Queue__jki_lib_state_machine.vi"("State(s) in (\"\")"=w1327) -> ("States Out"=w1326:string)  [unwired: 14 in]
          }
          event Value Change {
            n698 = event-data() -> ("NewVal"=w1342:bool)  [unwired: 1 in, 2 out]
            n699 = case shown="False" w1342 {
              tunnel: w1345 -> [_ w1358]
              tunnel: w1344 -> [w1348 w1356]
              tunnel: [w1348 w1355] -> w1343
              tunnel: w1342 -> [_ w1353]
              frame False {
              }
              frame True {
                n700 = local read "Number of ON/OFF Cycles"() -> (w1350:i32)
                n701 = local read "Valve ON Time (mS)"() -> (w1349:u32)
                n702 = local read "Agilent Semaphore"() -> (w1359:T1[])
                n703 = Unbundle By Name(w1358) -> ("Agilent Switches"=w1357:T2[])
                n704 = local read "Test Type"() -> (w1351:T12)
                n705 = Number To Decimal String(number=6) -> (decimal integer string=w1361:string)  [unwired: 1 in]
                n706 = Not(x=w1353) -> (.not. x?=w1360:bool)
                n707 = call "WILT Agilent Valve Control.vi"("Station In"=w1361, "Agilent Channels In"=w1357, "Semaphore"=w1359, "Search"=T19 "Start Button", "Open/Close (F:Close)"=w1360, "error in (no error)"=w1356, "Test Type"=w1351, "Number Of Cycles"=w1350, "Cycle Time (mS)"=w1349) -> ("error out"=w1355:errorcluster)  [unwired: 4 in, 2 out]
              }
            }
            n708 = call <vilib>:"Add State(s) to Queue__jki_lib_state_machine.vi"("State(s) in (\"\")"=w1347) -> ("States Out"=w1346:string)  [unwired: 14 in]
          }
          event Value Change {
            n709 = event-data() -> ("NewVal"=w1362:bool)  [unwired: 1 in, 2 out]
            n710 = case shown="True" w1362 {
              tunnel: w1365 -> [_ w1378]
              tunnel: w1364 -> [w1368 w1376]
              tunnel: [w1368 w1375] -> w1363
              tunnel: w1362 -> [_ w1373]
              frame False {
              }
              frame True {
                n711 = local read "Number of ON/OFF Cycles"() -> (w1370:i32)
                n712 = local read "Valve ON Time (mS)"() -> (w1369:u32)
                n713 = local read "Agilent Semaphore"() -> (w1379:T1[])
                n714 = Unbundle By Name(w1378) -> ("Agilent Switches"=w1377:T2[])
                n715 = local read "Test Type"() -> (w1371:T12)
                n716 = Number To Decimal String(number=7) -> (decimal integer string=w1381:string)  [unwired: 1 in]
                n717 = Not(x=w1373) -> (.not. x?=w1380:bool)
                n718 = call "WILT Agilent Valve Control.vi"("Station In"=w1381, "Agilent Channels In"=w1377, "Semaphore"=w1379, "Search"=T19 "Start Button", "Open/Close (F:Close)"=w1380, "error in (no error)"=w1376, "Test Type"=w1371, "Number Of Cycles"=w1370, "Cycle Time (mS)"=w1369) -> ("error out"=w1375:errorcluster)  [unwired: 4 in, 2 out]
              }
            }
            n719 = call <vilib>:"Add State(s) to Queue__jki_lib_state_machine.vi"("State(s) in (\"\")"=w1367) -> ("States Out"=w1366:string)  [unwired: 14 in]
          }
          event Value Change {
            n720 = event-data() -> ("NewVal"=w1382:bool)  [unwired: 1 in, 2 out]
            n721 = case shown="True" w1382 {
              tunnel: w1385 -> [_ w1398]
              tunnel: w1384 -> [w1388 w1396]
              tunnel: [w1388 w1395] -> w1383
              tunnel: w1382 -> [_ w1393]
              frame False {
              }
              frame True {
                n722 = local read "Number of ON/OFF Cycles"() -> (w1390:i32)
                n723 = local read "Valve ON Time (mS)"() -> (w1389:u32)
                n724 = local read "Agilent Semaphore"() -> (w1399:T1[])
                n725 = Unbundle By Name(w1398) -> ("Agilent Switches"=w1397:T2[])
                n726 = local read "Test Type"() -> (w1391:T12)
                n727 = Number To Decimal String(number=8) -> (decimal integer string=w1401:string)  [unwired: 1 in]
                n728 = Not(x=w1393) -> (.not. x?=w1400:bool)
                n729 = call "WILT Agilent Valve Control.vi"("Station In"=w1401, "Agilent Channels In"=w1397, "Semaphore"=w1399, "Search"=T19 "Start Button", "Open/Close (F:Close)"=w1400, "error in (no error)"=w1396, "Test Type"=w1391, "Number Of Cycles"=w1390, "Cycle Time (mS)"=w1389) -> ("error out"=w1395:errorcluster)  [unwired: 4 in, 2 out]
              }
            }
            n730 = call <vilib>:"Add State(s) to Queue__jki_lib_state_machine.vi"("State(s) in (\"\")"=w1387) -> ("States Out"=w1386:string)  [unwired: 14 in]
          }
          event Value Change {
            n731 = event-data() -> ("NewVal"=w1402:bool)  [unwired: 1 in, 2 out]
            n732 = case shown="False" w1402 {
              tunnel: w1405 -> [_ w1418]
              tunnel: w1404 -> [w1408 w1416]
              tunnel: [w1408 w1415] -> w1403
              tunnel: w1402 -> [_ w1413]
              frame False {
              }
              frame True {
                n733 = local read "Number of ON/OFF Cycles"() -> (w1410:i32)
                n734 = local read "Valve ON Time (mS)"() -> (w1409:u32)
                n735 = local read "Agilent Semaphore"() -> (w1419:T1[])
                n736 = Unbundle By Name(w1418) -> ("Agilent Switches"=w1417:T2[])
                n737 = local read "Test Type"() -> (w1411:T12)
                n738 = Number To Decimal String(number=9) -> (decimal integer string=w1421:string)  [unwired: 1 in]
                n739 = Not(x=w1413) -> (.not. x?=w1420:bool)
                n740 = call "WILT Agilent Valve Control.vi"("Station In"=w1421, "Agilent Channels In"=w1417, "Semaphore"=w1419, "Search"=T19 "Start Button", "Open/Close (F:Close)"=w1420, "error in (no error)"=w1416, "Test Type"=w1411, "Number Of Cycles"=w1410, "Cycle Time (mS)"=w1409) -> ("error out"=w1415:errorcluster)  [unwired: 4 in, 2 out]
              }
            }
            n741 = call <vilib>:"Add State(s) to Queue__jki_lib_state_machine.vi"("State(s) in (\"\")"=w1407) -> ("States Out"=w1406:string)  [unwired: 14 in]
          }
          event Value Change {
            n742 = event-data() -> ("NewVal"=w1422:bool)  [unwired: 1 in, 2 out]
            n743 = case shown="False" w1422 {
              tunnel: w1425 -> [_ w1438]
              tunnel: w1424 -> [w1428 w1436]
              tunnel: [w1428 w1435] -> w1423
              tunnel: w1422 -> [_ w1433]
              frame False {
              }
              frame True {
                n744 = local read "Number of ON/OFF Cycles"() -> (w1430:i32)
                n745 = local read "Valve ON Time (mS)"() -> (w1429:u32)
                n746 = local read "Agilent Semaphore"() -> (w1439:T1[])
                n747 = Unbundle By Name(w1438) -> ("Agilent Switches"=w1437:T2[])
                n748 = local read "Test Type"() -> (w1431:T12)
                n749 = Number To Decimal String(number=10) -> (decimal integer string=w1441:string)  [unwired: 1 in]
                n750 = Not(x=w1433) -> (.not. x?=w1440:bool)
                n751 = call "WILT Agilent Valve Control.vi"("Station In"=w1441, "Agilent Channels In"=w1437, "Semaphore"=w1439, "Search"=T19 "Start Button", "Open/Close (F:Close)"=w1440, "error in (no error)"=w1436, "Test Type"=w1431, "Number Of Cycles"=w1430, "Cycle Time (mS)"=w1429) -> ("error out"=w1435:errorcluster)  [unwired: 4 in, 2 out]
              }
            }
            n752 = call <vilib>:"Add State(s) to Queue__jki_lib_state_machine.vi"("State(s) in (\"\")"=w1427) -> ("States Out"=w1426:string)  [unwired: 14 in]
          }
          event Value Change {
            n753 = event-data() -> ("NewVal"=w1442:bool)  [unwired: 1 in, 2 out]
            n754 = case shown="True" w1442 {
              tunnel: w1445 -> [_ w1458]
              tunnel: w1444 -> [w1448 w1456]
              tunnel: [w1448 w1455] -> w1443
              tunnel: w1442 -> [_ w1453]
              frame False {
              }
              frame True {
                n755 = local read "Number of ON/OFF Cycles"() -> (w1450:i32)
                n756 = local read "Valve ON Time (mS)"() -> (w1449:u32)
                n757 = local read "Agilent Semaphore"() -> (w1459:T1[])
                n758 = Unbundle By Name(w1458) -> ("Agilent Switches"=w1457:T2[])
                n759 = local read "Test Type"() -> (w1451:T12)
                n760 = Number To Decimal String(number=11) -> (decimal integer string=w1461:string)  [unwired: 1 in]
                n761 = Not(x=w1453) -> (.not. x?=w1460:bool)
                n762 = call "WILT Agilent Valve Control.vi"("Station In"=w1461, "Agilent Channels In"=w1457, "Semaphore"=w1459, "Search"=T19 "Start Button", "Open/Close (F:Close)"=w1460, "error in (no error)"=w1456, "Test Type"=w1451, "Number Of Cycles"=w1450, "Cycle Time (mS)"=w1449) -> ("error out"=w1455:errorcluster)  [unwired: 4 in, 2 out]
              }
            }
            n763 = call <vilib>:"Add State(s) to Queue__jki_lib_state_machine.vi"("State(s) in (\"\")"=w1447) -> ("States Out"=w1446:string)  [unwired: 14 in]
          }
          event Value Change {
            n764 = event-data() -> ("NewVal"=w1462:bool)  [unwired: 1 in, 2 out]
            n765 = case shown="False" w1462 {
              tunnel: w1465 -> [_ w1478]
              tunnel: w1464 -> [w1468 w1476]
              tunnel: [w1468 w1475] -> w1463
              tunnel: w1462 -> [_ w1473]
              frame False {
              }
              frame True {
                n766 = local read "Number of ON/OFF Cycles"() -> (w1470:i32)
                n767 = local read "Valve ON Time (mS)"() -> (w1469:u32)
                n768 = local read "Agilent Semaphore"() -> (w1479:T1[])
                n769 = Unbundle By Name(w1478) -> ("Agilent Switches"=w1477:T2[])
                n770 = local read "Test Type"() -> (w1471:T12)
                n771 = Number To Decimal String(number=12) -> (decimal integer string=w1481:string)  [unwired: 1 in]
                n772 = Not(x=w1473) -> (.not. x?=w1480:bool)
                n773 = call "WILT Agilent Valve Control.vi"("Station In"=w1481, "Agilent Channels In"=w1477, "Semaphore"=w1479, "Search"=T19 "Start Button", "Open/Close (F:Close)"=w1480, "error in (no error)"=w1476, "Test Type"=w1471, "Number Of Cycles"=w1470, "Cycle Time (mS)"=w1469) -> ("error out"=w1475:errorcluster)  [unwired: 4 in, 2 out]
              }
            }
            n774 = call <vilib>:"Add State(s) to Queue__jki_lib_state_machine.vi"("State(s) in (\"\")"=w1467) -> ("States Out"=w1466:string)  [unwired: 14 in]
          }
          event Value Change {
            n775 = event-data() -> ("NewVal"=w1482:bool)  [unwired: 1 in, 2 out]
            n776 = case shown="False" w1482 {
              tunnel: w1485 -> [_ w1498]
              tunnel: w1484 -> [w1488 w1496]
              tunnel: [w1488 w1495] -> w1483
              tunnel: w1482 -> [_ w1493]
              frame False {
              }
              frame True {
                n777 = local read "Number of ON/OFF Cycles"() -> (w1490:i32)
                n778 = local read "Valve ON Time (mS)"() -> (w1489:u32)
                n779 = local read "Agilent Semaphore"() -> (w1499:T1[])
                n780 = Unbundle By Name(w1498) -> ("Agilent Switches"=w1497:T2[])
                n781 = local read "Test Type"() -> (w1491:T12)
                n782 = Number To Decimal String(number=13) -> (decimal integer string=w1501:string)  [unwired: 1 in]
                n783 = Not(x=w1493) -> (.not. x?=w1500:bool)
                n784 = call "WILT Agilent Valve Control.vi"("Station In"=w1501, "Agilent Channels In"=w1497, "Semaphore"=w1499, "Search"=T19 "Start Button", "Open/Close (F:Close)"=w1500, "error in (no error)"=w1496, "Test Type"=w1491, "Number Of Cycles"=w1490, "Cycle Time (mS)"=w1489) -> ("error out"=w1495:errorcluster)  [unwired: 4 in, 2 out]
              }
            }
            n785 = call <vilib>:"Add State(s) to Queue__jki_lib_state_machine.vi"("State(s) in (\"\")"=w1487) -> ("States Out"=w1486:string)  [unwired: 14 in]
          }
          event Value Change {
            n786 = event-data() -> ("NewVal"=w1502:bool)  [unwired: 1 in, 2 out]
            n787 = case shown="True" w1502 {
              tunnel: w1505 -> [_ w1518]
              tunnel: w1504 -> [w1508 w1516]
              tunnel: [w1508 w1515] -> w1503
              tunnel: w1502 -> [_ w1513]
              frame False {
              }
              frame True {
                n788 = local read "Number of ON/OFF Cycles"() -> (w1510:i32)
                n789 = local read "Valve ON Time (mS)"() -> (w1509:u32)
                n790 = local read "Agilent Semaphore"() -> (w1519:T1[])
                n791 = Unbundle By Name(w1518) -> ("Agilent Switches"=w1517:T2[])
                n792 = local read "Test Type"() -> (w1511:T12)
                n793 = Number To Decimal String(number=14) -> (decimal integer string=w1521:string)  [unwired: 1 in]
                n794 = Not(x=w1513) -> (.not. x?=w1520:bool)
                n795 = call "WILT Agilent Valve Control.vi"("Station In"=w1521, "Agilent Channels In"=w1517, "Semaphore"=w1519, "Search"=T19 "Start Button", "Open/Close (F:Close)"=w1520, "error in (no error)"=w1516, "Test Type"=w1511, "Number Of Cycles"=w1510, "Cycle Time (mS)"=w1509) -> ("error out"=w1515:errorcluster)  [unwired: 4 in, 2 out]
              }
            }
            n796 = call <vilib>:"Add State(s) to Queue__jki_lib_state_machine.vi"("State(s) in (\"\")"=w1507) -> ("States Out"=w1506:string)  [unwired: 14 in]
          }
          event Value Change {
            n797 = event-data() -> ("NewVal"=w1522:bool)  [unwired: 1 in, 2 out]
            n798 = case shown="True" w1522 {
              tunnel: w1525 -> [_ w1538]
              tunnel: w1524 -> [w1528 w1536]
              tunnel: [w1528 w1535] -> w1523
              tunnel: w1522 -> [_ w1533]
              frame False {
              }
              frame True {
                n799 = local read "Number of ON/OFF Cycles"() -> (w1530:i32)
                n800 = local read "Valve ON Time (mS)"() -> (w1529:u32)
                n801 = local read "Agilent Semaphore"() -> (w1539:T1[])
